vi "gaussian correlation time.vi"() -> ()   [LabVIEW 2014]
uses:
  <vilib>/userdefined/High Color/IMAQdx.ctl
  <vilib>/Utility/file.llb/Write To Spreadsheet File (DBL).vi
  <vilib>/vision/driver/NI_Vision_Acquisition_Software.lvlib
panel:
  in  "Tags":string
  in  "Wait before recording (s)":dbl
  in  "Correlation Time (s)":dbl
  in  "Start Recording":bool
  in  "Max Power (uW/mm^2)":dbl
  in  "Min Power (uW/mm^2)":dbl
  in  "Frames":i32
  in  "Sigma (uW/mm^2)":dbl
  in  "Offset Power (uW/mm^2)":dbl
  out "Error":string
  out "Save Directory":path
  out "Buffer Number Out":u32
  out "Image":T1(plugin-control)
  in  "stop":bool
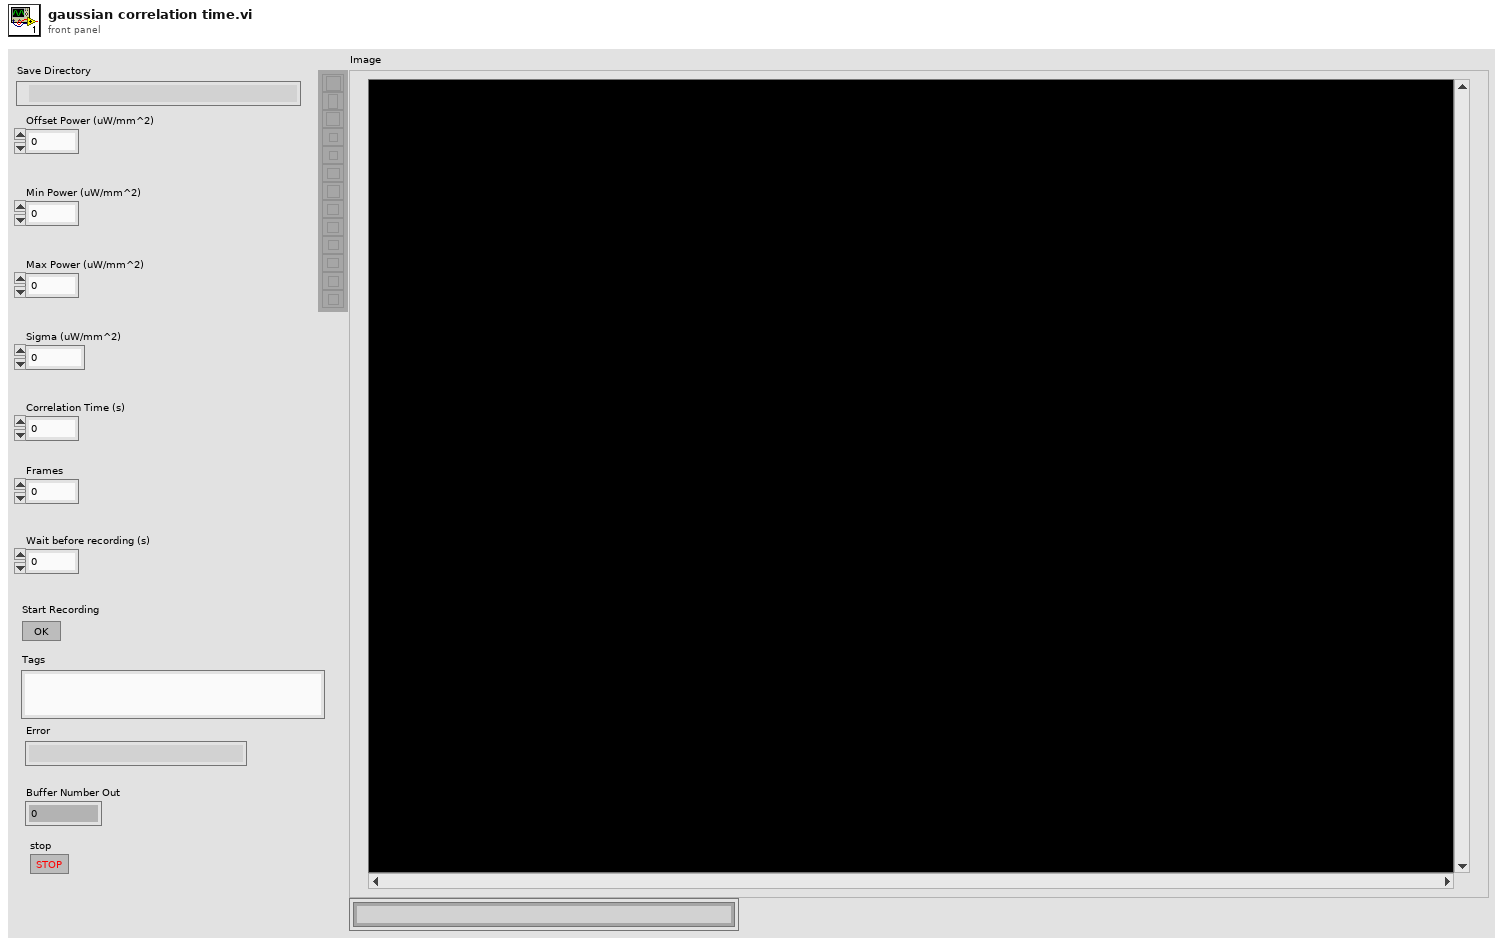
[diagram p1: front panel]
types:
  T1 = typedef "IMAQ Image.ctl" = refnum<image>
  T2 = typedef "IMAQdx.ctl" = refnum<k21>
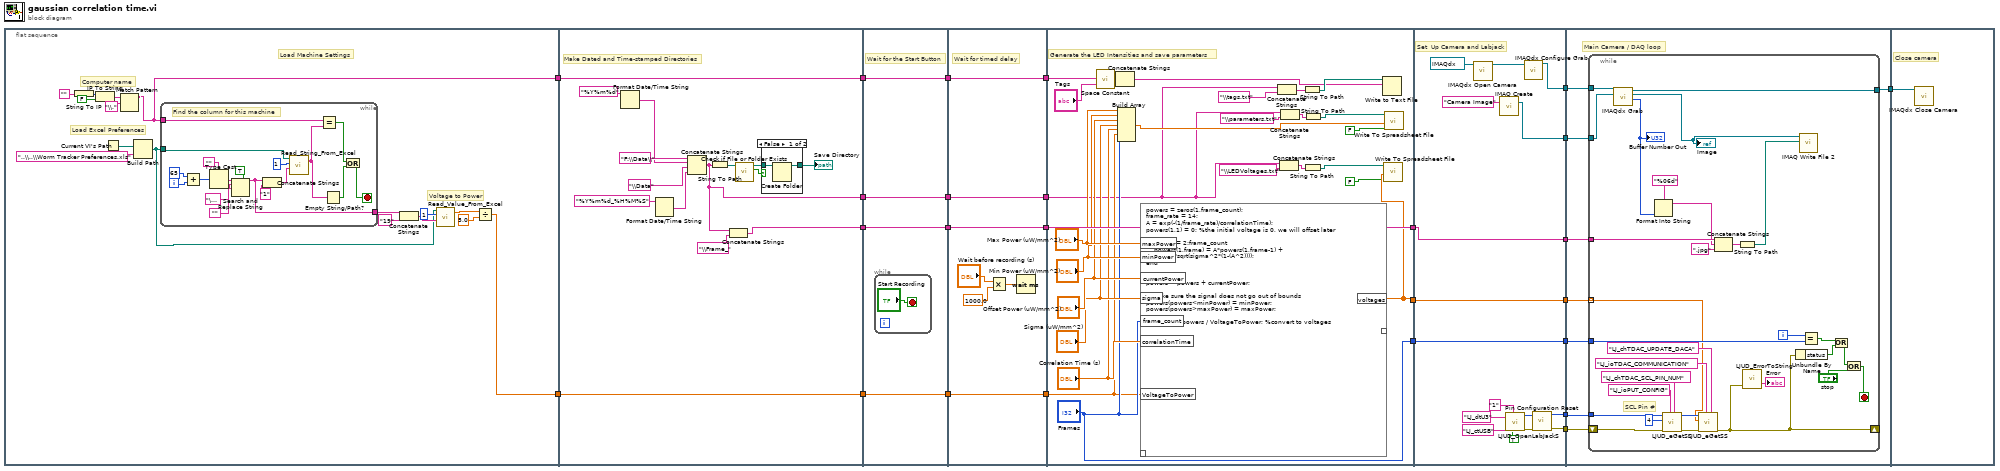
[diagram p0: block diagram]
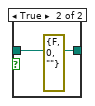
[diagram p2: hidden frame]
diagram:
  n1 = flat-sequence {
    tunnel: [w27] -> w5
    tunnel: [w26] -> w1
    tunnel: [w64] -> w14
    tunnel: [w62] -> w13
    tunnel: [w61] -> w6
    tunnel: w5 -> [w61]
    tunnel: [w60] -> w2
    tunnel: w1 -> [w60]
    tunnel: w14 -> [w81]
    tunnel: [w81] -> w12
    tunnel: w13 -> [w80]
    tunnel: [w80] -> w10
    tunnel: [w79] -> w7
    tunnel: w6 -> [w79]
    tunnel: [w78] -> w3
    tunnel: w2 -> [w78]
    tunnel: w12 -> [w89]
    tunnel: [w89] -> w11
    tunnel: w10 -> [w88]
    tunnel: [w88] -> w9
    tunnel: [w84] -> w8
    tunnel: w7 -> [w84]
    tunnel: [w83] -> w4
    tunnel: w3 -> [w83]
    tunnel: w11 -> [w113]
    tunnel: [w113] -> w19
    tunnel: [w111] -> w17
    tunnel: ["Frames"] -> w16
    tunnel: w9 -> [w97]
    tunnel: w8 -> [w98]
    tunnel: w4 -> [w93]
    tunnel: w19 -> [w126]
    tunnel: [w128] -> w25
    tunnel: [w127] -> w24
    tunnel: [w126] -> w23
    tunnel: [w118] -> w21
    tunnel: [w117] -> w20
    tunnel: [w122] -> w18
    tunnel: w17 -> [w122]
    tunnel: w16 -> [w121]
    tunnel: [w121] -> w15
    tunnel: w25 -> [w139]
    tunnel: w24 -> [w138]
    tunnel: w23 -> [w137]
    tunnel: [w136] -> w22
    tunnel: w21 -> [w135]
    tunnel: w20 -> [w134]
    tunnel: w18 -> [w133]
    tunnel: w15 -> [w132]
    tunnel: w22 -> [w170]
    frame #0 {
      # "Voltage to Power"
      # "Load Excel Preferences"
      # "Computer name"
      # "Load Machine Settings"
      n2 = String To IP(1:"") -> (0:w41:u32)
      n3 = IP To String(1:FALSE, 2:w41) -> (0:w38:string)
      n4 = Current VI's Path() -> (path=w36:path)
      n5 = Match Pattern(string=w38, regular expression="\\.") -> (before substring=w26:string)  [unwired: 1 in, 3 out]
      n6 = Build Path(base path=w36, name or relative path="..\\..\\Worm Tracker Preferences.xls") -> (appended path=w30:path)
      n7 = while {
        tunnel: w30 -> [w54]
        tunnel: w26 -> [w51]
        tunnel: [w42] -> w34
        i -> [w59]
        stop <- w48 stop-if-true
        # "Find the column for this machine"
        n8 = Add(x=65, y=w59) -> (x+y=w57:i32)
        n9 = Type Cast(type="", x=w57) -> (*(type *) &x=w43:string)
        n10 = Search and Replace String(replace all?=TRUE, input string=w43, search string="\u0000", replace string="") -> (result string=w42:string)  [unwired: 4 in, 3 out]
        n11 = Concatenate Strings(w42, "1") -> (w53:string)
        n12 = call "Read_String_From_Excel.vi"("Selected Cell"=w53, "Work Sheet"=1, "Excel File Path"=w54) -> ("Data from Cell"=w52:string)  [unwired: 1 in, 1 out]
        n13 = Equal?(x=w51, y=w52) -> (x = y?=w50:bool)
        n14 = Empty String/Path?(string/path=w52) -> (empty?=w49:bool)
        n15 = Or(x=w50, y=w49) -> (x .or. y?=w48:bool)
      }
      n16 = Concatenate Strings(w34, "19") -> (w32:string)
      n17 = call "Read_Value_From_Excel.vi"("Selected Cell"=w32, "Work Sheet"=1, "Excel File Path"=w30) -> ("Data from Cell"=w29:dbl)  [unwired: 1 in, 1 out]
      n18 = Divide(x=w29, y=5.0) -> (x/y=w27:dbl)
    }
    frame #1 {
      # "Make Dated and Time-stamped Directories"
      n19 = Format Date/Time String(time format string (%c)="%Y%m%d") -> (date/time string=w65:string)  [unwired: 2 in]
      n20 = Format Date/Time String(time format string (%c)="%Y%m%d_%H%M%S") -> (date/time string=w69:string)  [unwired: 2 in]
      n21 = Concatenate Strings("F:\\Data\\", w65, "\\Data", w69) -> (w62:string)
      n22 = String To Path(string=w62) -> (path=w68:path)
      n23 = Concatenate Strings(w62, "\\Frame_") -> (w64:string)
      n24 = call <vilib>:"Check if File or Folder Exists.vi"("path"=w68) -> ("file or folder exists?"=w73:bool, "dup path"=w72:path)  [unwired: 8 in, 1 out]
      n25 = case shown="False" w73 {
        tunnel: [w75 w77] -> w67
        tunnel: w72 -> [w76 w77]
        frame False {
          n26 = Create Folder(path (use dialog)=w76) -> (created path=w75:path)  [unwired: 2 in, 2 out]
        }
        frame True {
          (unwired) errorcluster {"status"=FALSE, "code"=0, "source"=""} ("error out")
        }
      }
      "Save Directory" <- w67
    }
    frame #2 {
      # "Wait for the Start Button"
      n27 = while {
        stop <- "Start Recording" stop-if-true
      }
    }
    frame #3 {
      # "Wait for timed delay"
      n28 = Multiply(x="Wait before recording (s)", y=1000.0) -> (x*y=w86:dbl)
      n29 = Wait (ms)(milliseconds to wait=w86) -> ()  [unwired: 1 out]
    }
    frame #4 {
      # "Generate the LED Intensities and save parameters"
      n30 = call <vilib>:"Space Constant.vi"() -> ("String"=w91:string)
      n31 = Concatenate Strings(w93, w91, "Tags") -> (w90:string)
      n32 = Build Array("Max Power (uW/mm^2)", "Min Power (uW/mm^2)", "Offset Power (uW/mm^2)", "Sigma (uW/mm^2)", "Correlation Time (s)", w98, "Frames") -> (w101:dbl[])
      n33 = script code="powers = zeros(1,frame_count);\nframe_rate = 14;\nA = exp(-(1/frame_rate)/correlationTime);\npowers(1,1) = 0; %the initial voltage is 0, we will offset later\n\nfor frame = 2:frame_count\n    powers(1,frame) = A*powers(1,frame-1) + (randn(1)*sqrt(sigma^2*(1-(A^2))));\nend\n\n%offset\npowers = powers + currentPower;\n\n%make sure the signal does not go out of bounds\npowers(powers<minPower) = minPower;\npowers(powers>maxPower) = maxPower;\n\nvoltages = powers / VoltageToPower; %convert to voltages"("currentPower"="Offset Power (uW/mm^2)", "frame_count"="Frames", "sigma"="Sigma (uW/mm^2)", "minPower"="Min Power (uW/mm^2)", "maxPower"="Max Power (uW/mm^2)", "correlationTime"="Correlation Time (s)", "VoltageToPower"=w98) -> ("voltages"=w111:dbl[])  [unwired: 1 in, 1 out]
      n34 = Concatenate Strings(w97, "\\tags.txt") -> (w95:string)
      n35 = Concatenate Strings(w97, "\\LEDVoltages.txt") -> (w115:string)
      n36 = Concatenate Strings(w97, "\\parameters.txt") -> (w105:string)
      n37 = String To Path(string=w95) -> (path=w94:path)
      n38 = String To Path(string=w115) -> (path=w114:path)
      n39 = String To Path(string=w105) -> (path=w104:path)
      n40 = Write to Text File(file (use dialog)=w94, text=w90) -> ()  [unwired: 2 in, 3 out]
      n41 = call-poly <vilib>:"Write To Spreadsheet File.vi"("append to file? (new file:F)"=FALSE, "1D data"=w111, "file path (dialog if empty)"=w114) -> ()  [unwired: 5 in, 1 out]
      n42 = call-poly <vilib>:"Write To Spreadsheet File.vi"("append to file? (new file:F)"=FALSE, "1D data"=w101, "file path (dialog if empty)"=w104) -> ()  [unwired: 5 in, 1 out]
    }
    frame #5 {
      # "Set  Up Camera and Labjack"
      n43 = call <vilib>:"IMAQdx Open Camera.vi"("Session In"=T2 "cam0") -> ("Session Out"=w130:T2)  [unwired: 9 in, 1 out]
      n44 = call "IMAQ Create"("Image Name"="Camera Image") -> ("New Image"=w127:T1)  [unwired: 4 in, 1 out]
      n45 = call "LJUD_OpenLabJackS.vi"("FirstFound"=TRUE, "Address"="1" ("DeviceType"), "ConnectionType"="LJ_ctUSB", "DeviceType"="LJ_dtU3") -> ("error out"=w116:errorcluster, "Handle"=w119:i32)  [unwired: 5 in, 1 out]
      n46 = call <vilib>:"IMAQdx Configure Grab.vi"("Session In"=w130) -> ("Session Out"=w128:T2)  [unwired: 9 in, 1 out]
      n47 = call "Pin Configuration Reset.vi"("error in"=w116, "Handle In"=w119) -> ("error out"=w117:errorcluster, "Handle Out"=w118:i32)  [unwired: 8 in]
    }
    frame #6 {
      # "Main Camera / DAQ loop"
      n48 = while {
        tunnel: w139 -> [w169]
        tunnel: [w168] -> w136
        tunnel: w138 -> [w167]
        tunnel: w137 -> [w165]
        tunnel: w135 -> [w142]
        shift-right: [w143] -> _
        shift-left: w134 -> [w141]
        tunnel: w133 -> [w140] mode=indexing
        tunnel: w132 -> [w151]
        i -> [w152]
        stop <- w158 stop-if-true
        # "SCL Pin #"
        n49 = call <vilib>:"IMAQdx Grab.vi"("Image In"=w167, "Session In"=w169) -> ("Buffer Number Out"=w161:u32, "Image Out"=w166:T1, "Session Out"=w168:T2)  [unwired: 6 in, 1 out]
        "Image" <- w166
        "Buffer Number Out" <- w161
        n50 = Format Into String(format string="%06d" ("string"), w161) -> (resulting string=w160:string)  [unwired: 2 in, 1 out]
        n51 = call "LJUD_eGetSS.vi"("Channel"="LJ_chTDAC_SCL_PIN_NUM", "IOType"="LJ_ioPUT_CONFIG", "error in"=w141, "Value Write"=4, "Handle In"=w142) -> ("error out"=w144:errorcluster, "Handle Out"=w147:i32)  [unwired: 4 in, 1 out]
        n52 = call "LJUD_eGetSS.vi"("Channel"="LJ_chTDAC_UPDATE_DACA", "IOType"="LJ_ioTDAC_COMMUNICATION", "error in"=w144, "Value Write"=w140, "Handle In"=w147) -> ("error out"=w143:errorcluster)  [unwired: 4 in, 2 out]
        n53 = Concatenate Strings(w165, w160, ".jpg" ("string")) -> (w163:string)
        n54 = String To Path(string=w163) -> (path=w162:path)
        n55 = call "LJUD_ErrorToString.vi"("error in"=w143) -> ("String"=→"Error":string)  [unwired: 10 in]
        n56 = Unbundle By Name(w143) -> ("status"=w155:bool)
        n57 = call-poly "IMAQ Write File 2"("File Path"=w162, "Image"=w166) -> ()  [unwired: 8 in, 2 out]
        n58 = Equal?(x=w152, y=w151) -> (x = y?=w154:bool)
        n59 = Or(x=w154, y=w155) -> (x .or. y?=w153:bool)
        n60 = Or(x=w153, y="stop") -> (x .or. y?=w158:bool)
      }
    }
    frame #7 {
      # "Close camera"
      n61 = call <vilib>:"IMAQdx Close Camera.vi"("Session In"=w170) -> ()  [unwired: 10 in, 1 out]
    }
  }
